vi "DRIVE ARRAY to 2x2 INDICATOR.vi"(0 "VELOCITIES":dbl[](array[numeric]), 5 "STEER ANGLES\n(deg)":dbl[](array[numeric])) -> (4 "Array out":cluster{"swerve":dbl, "V":dbl}[][](array[cluster]))   [LabVIEW 2023]
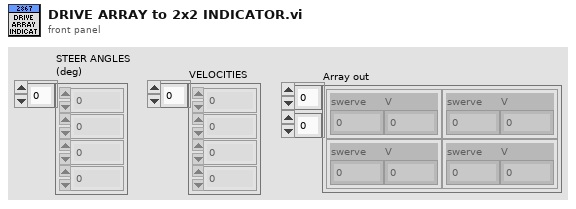
[diagram p1: front panel]
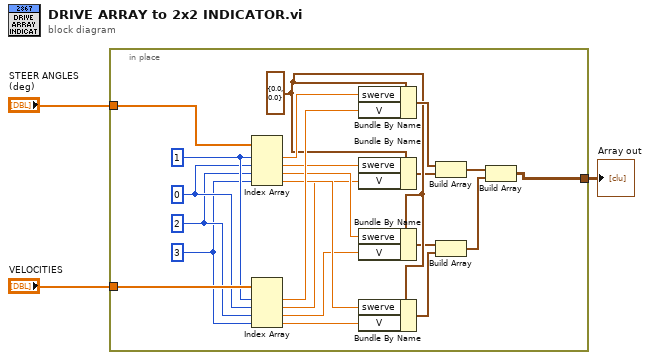
[diagram p0: block diagram]
diagram:
  n1 = in-place {
    in-place-border: "STEER ANGLES\n(deg)" -> [w23]
    in-place-border: "VELOCITIES" -> [w22]
    in-place-border: [w4] -> w3
    w8 = cluster{"swerve":dbl, "V":dbl} {"swerve"=0.0, "V"=0.0} ("Array 2")
    w18 = 3 ("index")
    w19 = 2 ("index")
    w20 = 0 ("index")
    w21 = 1 ("index")
    n2 = Index Array(array=w23, index #1=w21, index #2=w20, index #3=w19, index #4=w18) -> (element #1=w15:dbl, element #2=w14:dbl, element #3=w13:dbl, element #4=w12:dbl)
    n3 = Index Array(array=w22, index #1=w21, index #2=w20, index #3=w19, index #4=w18) -> (element #1=w16:dbl, element #2=w9:dbl, element #3=w10:dbl, element #4=w11:dbl)
    n4 = Bundle By Name(cluster=w8, "swerve"=w15, "V"=w16) -> (w17:cluster{"swerve":dbl, "V":dbl})
    n5 = Bundle By Name(cluster=w8, "swerve"=w14, "V"=w9) -> (w7:cluster{"swerve":dbl, "V":dbl})
    n6 = Bundle By Name(cluster=w8, "swerve"=w13, "V"=w10) -> (w6:cluster{"swerve":dbl, "V":dbl})
    n7 = Bundle By Name(cluster=w8, "swerve"=w12, "V"=w11) -> (w5:cluster{"swerve":dbl, "V":dbl})
    n8 = Build Array(w17, w7) -> (w25:cluster{"swerve":dbl, "V":dbl}[])
    n9 = Build Array(w6, w5) -> (w24:cluster{"swerve":dbl, "V":dbl}[])
    n10 = Build Array(w25, w24) -> (w4:cluster{"swerve":dbl, "V":dbl}[][])
  }
  "Array out" <- w3
